vi "Is Serial Info Valid.vi"(8 "Controller B":T1, 11 "Controller A":T1) -> (0 "B Valid?":bool, 1 "A Valid?":bool, 2 "Has Valid?":bool, 3 "Conflict?":bool)   [LabVIEW 2019, in "UI.lvlib"]
uses:
  Controller/Serial Info.ctl
  UI.lvlib
  Controller/Controller.lvlib
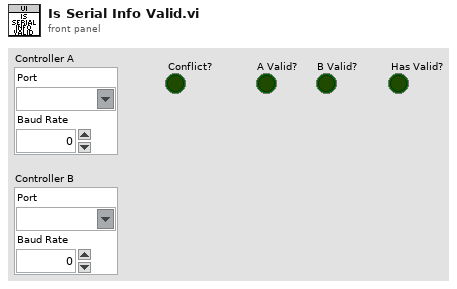
[diagram p1: front panel]
types:
  T1 = typedef "Controller.lvlib/Serial Info.ctl" = cluster{"Port":refnum<visa-resource-name>, "Baud Rate":u32}
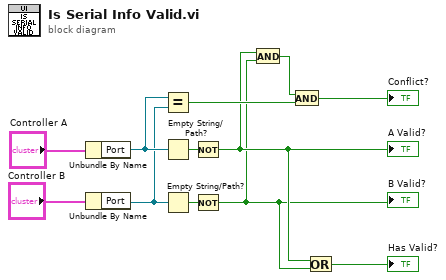
[diagram p0: block diagram]
diagram:
  n1 = Unbundle By Name("Controller A") -> ("Port"=w8:refnum<visa-resource-name>)
  n2 = Unbundle By Name("Controller B") -> ("Port"=w7:refnum<visa-resource-name>)
  n3 = Equal?(x=w8, y=w7) -> (x = y?=w6:bool)
  n4 = Empty String/Path?(string/path=w8) -> (empty?=w9:bool)
  n5 = Empty String/Path?(string/path=w7) -> (empty?=w10:bool)
  n6 = Not(x=w9) -> (.not. x?=w3:bool)
  "A Valid?" <- w3
  n7 = Not(x=w10) -> (.not. x?=w2:bool)
  "B Valid?" <- w2
  n8 = And(x=w3, y=w2) -> (x .and. y?=w4:bool)
  n9 = And(x=w4, y=w6) -> (x .and. y?=→"Conflict?":bool)
  n10 = Or(x=w3, y=w2) -> (x .or. y?=→"Has Valid?":bool)
